vi "Controller - State Process.vi"(8 "error in (no error)":errorcluster, 11 "View Model":T1) -> (0 "error out":errorcluster, 3 "View Model":T1)   [LabVIEW 2017]
doc: "Provide processing current state of Controller"
uses:
  Model/Controls/View Model.ctl
  Model/Controls/Shared Model.ctl
  Error Handler/Controls/Error Model.ctl
  Error Handler/Controls/Error Message.ctl
  Error Handler/Controls/Error Type.ctl
  Configuration/Controls/Config Model.ctl
  Configuration/Controls/Config DB Message.ctl
  Configuration/Controls/Config DB Command.ctl
  Configuration/Controls/Config DB Overhead.ctl
  Configuration/Controls/Config DB Record.ctl
  Controls/Controller Model.ctl
  Views/Vehicle Position Simulation View/Controls/Vehicle - Position.ctl
  Controls/Controller Overhead.ctl
  Controls/Controller Wash Step.ctl
  Controls/Controller State.ctl
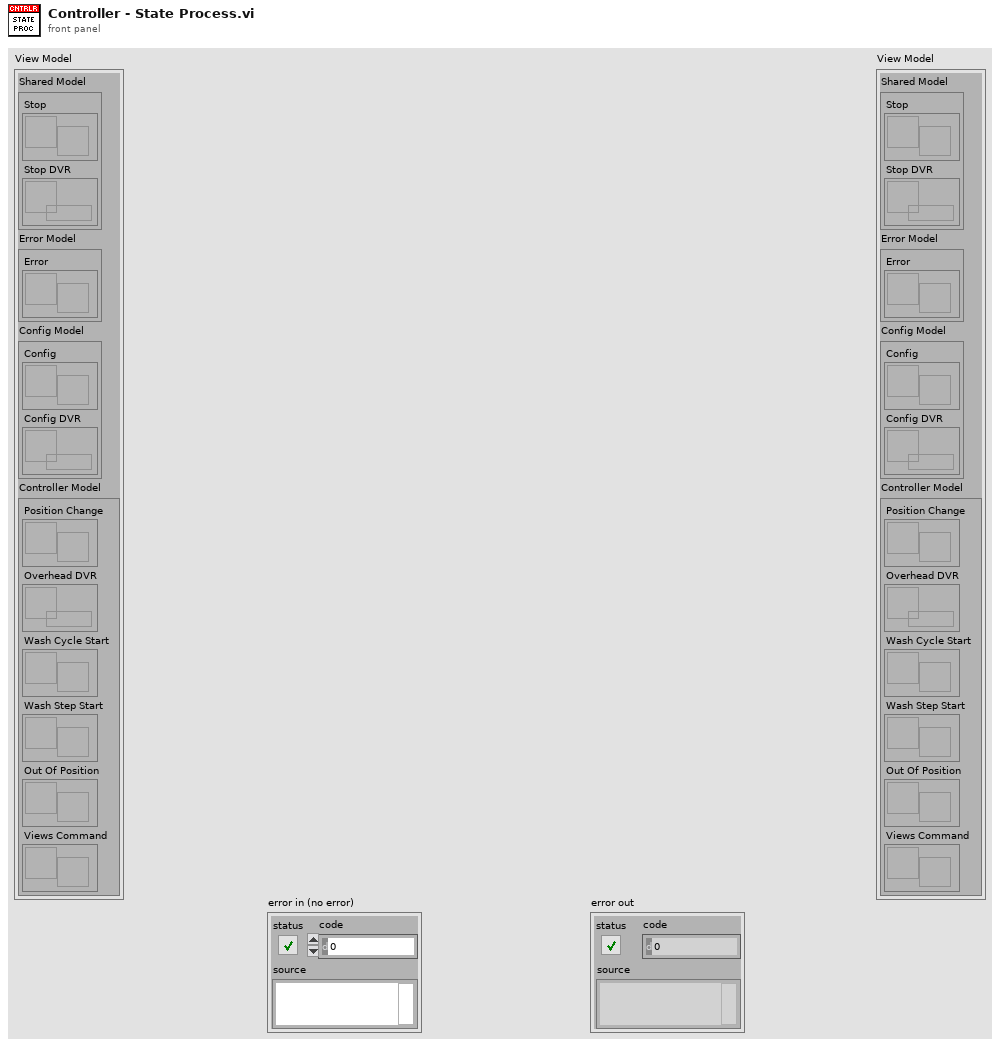
[diagram p1: front panel]
types:
  T1 = typedef "View Model.ctl" = cluster{"Shared Model":T2, "Error Model":T3, "Config Model":T4, "Controller Model":T5}
  T2 = typedef "Shared Model.ctl" = cluster{"Stop":refnum<user-event>, "Stop DVR":refnum<data-value>}
  T3 = typedef "Error Model.ctl" = cluster{"Error":refnum<user-event>}
  T4 = typedef "Config Model.ctl" = cluster{"Config":refnum<user-event>, "Config DVR":refnum<data-value>}
  T5 = typedef "Controller Model.ctl" = cluster{"Position Change":refnum<user-event>, "Overhead DVR":refnum<data-value>, "Wash Cycle Start":refnum<user-event>, "Wash Step Start":refnum<user-event>, "Out Of Position":refnum<user-event>, "Views Command":refnum<user-event>}
  T6 = typedef "Controller State.ctl" = enum16{"Initial", "Wait for Start", "Wash Cycle Start", "Wash Cycle Complete", "Wash Step Start", "Wash Step Execute", "Wash Step Complete", "Wait for Vehicle Position", "Wash Exit", "Wash Abort/Terminate"}
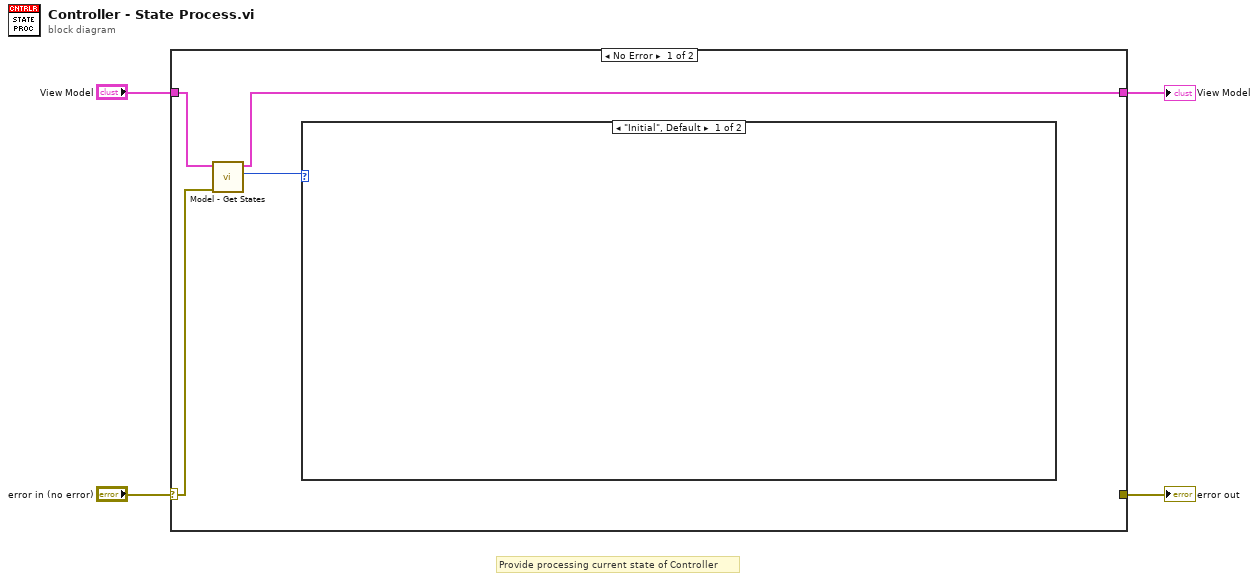
[diagram p0: block diagram]
diagram:
  # "Provide processing current state of Controller"
  n1 = case shown="No Error" "error in (no error)" {
    selector: "error in (no error)" -> [w7 w9]
    tunnel: "View Model" -> [w8 w10]
    tunnel: [_ w9] -> w2
    tunnel: [w5 w10] -> w1
    frame No Error {
      n2 = call "Model - Get States.vi"("error in (no error)"=w7, "View Model"=w8) -> ("Current State"=w6:T6, "View Model"=w5:T1)  [unwired: 6 in, 2 out]
      n3 = case shown="\"Initial\", Default" w6 {
        frame "Initial", Default {
        }
        frame "Wait for Start" {
        }
      }
    }
    frame Error {
    }
  }
  "View Model" <- w1
  "error out" <- w2
